vi "Set Select Event.vi"(8 "error in (no error)":errorcluster, 10 "Select App Event":refnum<user-event>, 11 "GWebAppArrayPanel in":refnum<class "GWebAppArrayPanel.lvclass">) -> (0 "error out":errorcluster, 3 "GWebAppArrayPanel out":refnum<class "GWebAppArrayPanel.lvclass">)   [LabVIEW 2020, in "PicoG-App.lvlib" / "GWebAppArrayPanel.lvclass"]
uses:
  GWebAppArrayPanel.lvclass
  ViaApp/ViaApp.lvclass
  GWebAppArrayPanel.lvclass/GWebAppArrayPanel.ctl
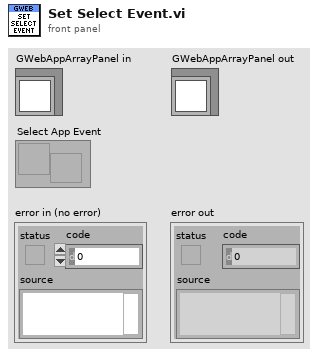
[diagram p1: front panel]
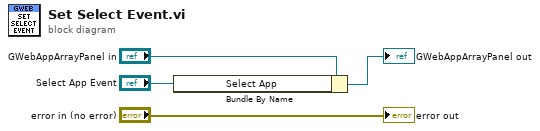
[diagram p0: block diagram]
diagram:
  n1 = Bundle By Name(cluster="GWebAppArrayPanel in", "Select App"="Select App Event") -> (→"GWebAppArrayPanel out":refnum<class "GWebAppArrayPanel.lvclass">)
  "error out" <- "error in (no error)"
